vi "Reset.vi"(8 "error in (no error)":errorcluster, 11 "VISA resource name":refnum<visa-resource-name>) -> (0 "error out":errorcluster, 3 "VISA resource name out":refnum<visa-resource-name>)   [LabVIEW 2012, in "ValveController.lvlib"]
doc: "Resets the instrument and then sends a set of default setup commands to the instrument."
uses:
  <instrlib>/ValveController/ValveController.lvlib
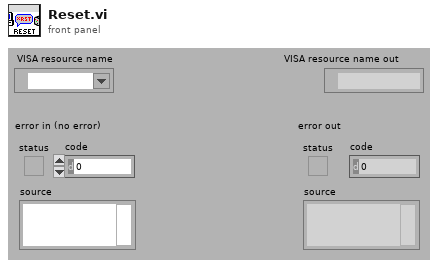
[diagram p1: front panel]
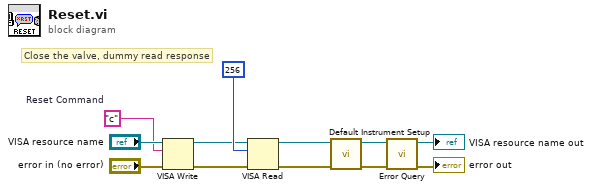
[diagram p0: block diagram]
diagram:
  w10 = "c"  # Reset Command
  # "Close the valve, dummy read response"
  n1 = VISA Write(VISA resource name="VISA resource name", write buffer=w10, error in (no error)="error in (no error)") -> (VISA resource name out=w4:refnum<visa-resource-name>, error out=w3:errorcluster)  [unwired: 1 out]
  n2 = VISA Read(VISA resource name=w4, byte count=u32 256, error in (no error)=w3) -> (VISA resource name out=w1:refnum<visa-resource-name>, error out=w2:errorcluster)  [unwired: 2 out]
  n3 = call <instrlib>:"Default Instrument Setup.vi"("error in (no error)"=w2, "VISA resource name"=w1) -> ("error out"=w9:errorcluster, "VISA resource name out"=w8:refnum<visa-resource-name>)  [unwired: 8 in]
  n4 = call <instrlib>:"Error Query.vi"("error in (no error)"=w9, "VISA resource name"=w8) -> ("error out"=→"error out":errorcluster, "VISA resource name out"=→"VISA resource name out":refnum<visa-resource-name>)  [unwired: 8 in]
